vi "flower_watering.vi"() -> ()   [LabVIEW 2021]
uses:
  <vilib>/Instr/_visa.llb/VISA Configure Serial Port (Instr).vi
panel:
  in  "stop":bool
  out "read buffer":string
  in  "byte count":u32
  in  "VISA resource name":refnum<visa-resource-name>
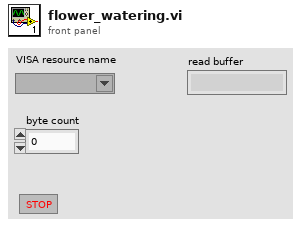
[diagram p1: front panel]
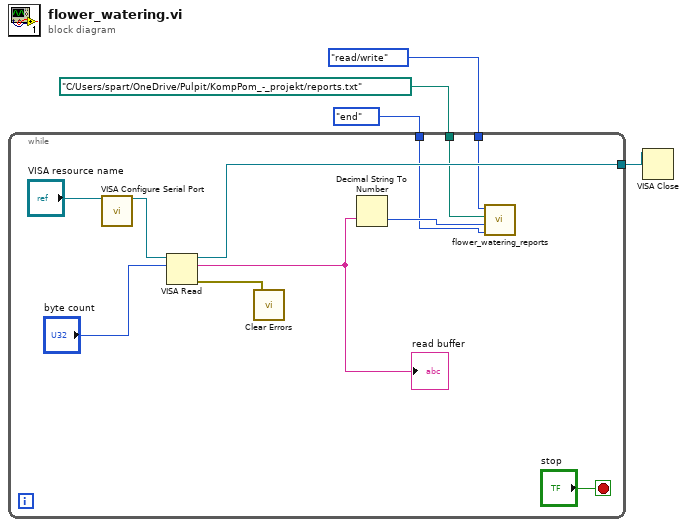
[diagram p0: block diagram]
diagram:
  n1 = while {
    tunnel: [w12] -> w4
    tunnel: path "C:/Users/spart/OneDrive/Pulpit/KompPom_-_projekt/reports.txt" ("Reports filepath") -> [w7]
    tunnel: enum16{"read/write", "read-only", "write-only"}."read/write" ("access (0:read/write)") -> [w6]
    tunnel: enum16{"start", "end", "current"}."end" ("from (0:start)") -> [w5]
    stop <- "stop" stop-if-true
    n2 = call-poly "VISA Configure Serial Port"("VISA resource name"="VISA resource name") -> ("VISA resource name out"=w13:refnum<visa-resource-name>)  [unwired: 13 in, 1 out]
    n3 = VISA Read(VISA resource name=w13, byte count="byte count") -> (VISA resource name out=w12:refnum<visa-resource-name>, read buffer=w10:string, error out=w9:errorcluster)  [unwired: 1 in, 1 out]
    "read buffer" <- w10
    n4 = call <vilib>:"Clear Errors.vi"("error in (no error)"=w9) -> ()  [unwired: 5 in, 2 out]
    n5 = Decimal String To Number(string=w10) -> (number=w8:i32)  [unwired: 2 in, 1 out]
    n6 = call "flower_watering_reports.vi"("from (0:start)"=w5, "Numeric"=w8, "Reports filepath"=w7, "access (0:read/write)"=w6) -> ()  [unwired: 1 in]
  }
  n7 = VISA Close(VISA resource name=w4) -> ()  [unwired: 1 in, 1 out]
